vi "Determine_Meas_Analysis.vi"(1 "Pre Setup String":string, 2 "Analysis info Cluster In":T1[](array[typedef]) {"Kurt_u" format="%_3g"; "u^4" format="%_3g"; "u^3" format="%_3g"; "Sd Error in Variance" format="%_3g"; "u^2" format="%_3g"; "Sd Error in Mean" format="%_3g"; "U" format="%_3g"; "Sync Delay Time (s)" format="%.4f"; "Total Meas Time (s)" format="%_5g"; "Skew_u" format="%_3g"; "% u'/U" format="%_3g"}) -> (0 "Analysis info Cluster Out":T1[](array[typedef]) {"Kurt_u" format="%_3g"; "u^4" format="%_3g"; "u^3" format="%_3g"; "Sd Error in Variance" format="%_3g"; "u^2" format="%_3g"; "Sd Error in Mean" format="%_3g"; "U" format="%_3g"; "Sync Delay Time (s)" format="%.4f"; "Total Meas Time (s)" format="%_5g"; "Skew_u" format="%_3g"; "% u'/U" format="%_3g"})   [LabVIEW 2022 SP3]
uses:
  Globals/Meas_global.vi
  Controls/Inst_type.ctl
  Controls/Analysis_info_cluster.ctl
  Controls/Instrument_Array.ctl
  Acquisition/PWA/PWAtasksGLOBAL.vi
  7 Hole Probe pressures to UVW/7HP_Global.vi
  Acquisition/Device ID port info.ctl
  Controls/channelState.ctl
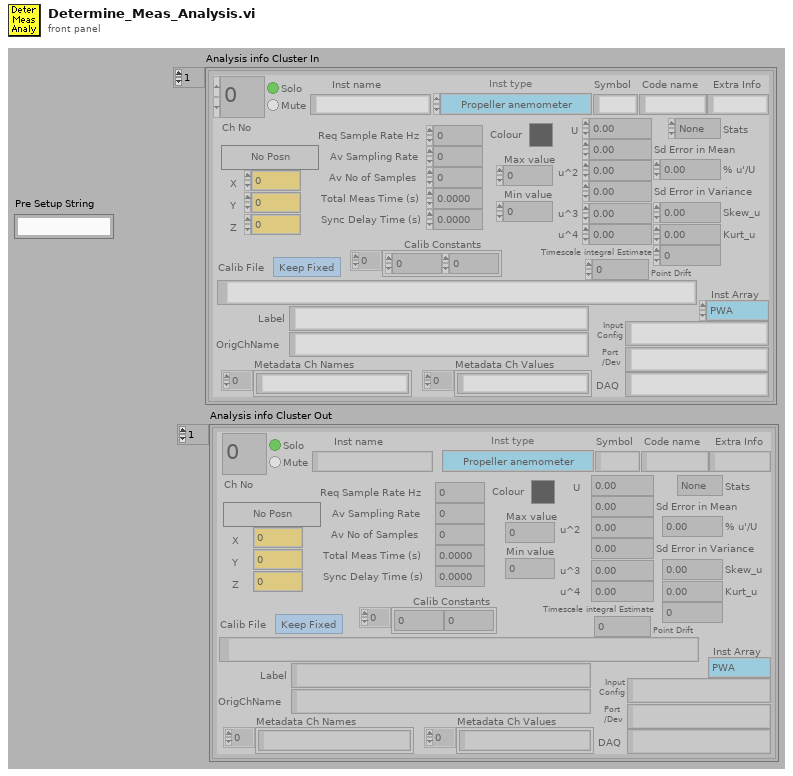
[diagram p1: front panel]
types:
  T1 = typedef "Analysis_info_cluster.ctl" = cluster{"Colour":u32, "Inst type":T2, "Inst name":string, "Symbol":string, "Code name":string, "Extra Info":string, "Inst Array":T3, "U":dbl, "u^2":dbl, "u^3":dbl, "u^4":dbl, "Skew_u":dbl, "Kurt_u":dbl, "Sd Error in Mean":dbl, "% u'/U":dbl, "X":dbl, "Y":dbl, "Z":dbl, "Timescale integral Estimate":dbl, "Sd Error in Variance":dbl, "Calib File":path, "Calib Constants":dbl[], "Output Position":bool, "Stats":enum16{"None", "Basic", "Full"}, "Av Sampling Rate":dbl, "Av No of Samples":dbl, "Total Meas Time (s)":dbl, "OrigChName":string, "Max value":dbl, "Min value":dbl, "Req Sample Rate Hz":dbl, "Sync Delay Time (s)":dbl, "Ch No":i16, "Device":string, "Use Latest Calib":bool, "Port":string, "Metadata Ch Names":string[], "Metadata Ch Values":string[], "Label":string, "chState":T4, "Point Drift":dbl, "inputConfig":string}
  T2 = typedef "Inst_type.ctl" = enum16{"Raw voltage", "Raw with zero offsetting", "Propeller anemometer", "Pressure Transducer", "Pitot-static tube", "Hot wire", "Cross wire 1", "Cross wire 2", "Generic Linear", "Generic Polynomial", "Generic BackPoly", "Fast FID", "Thermocouple", "Cold wire", "Pulsed Wire", "LDA Vel", "LDA Tran time", "LDA Arr time", "Microphone"}
  T3 = typedef "Instrument_Array.ctl" = enum16{"PWA", "LDA", "Analogue"}
  T4 = typedef "channelState.ctl" = enum32{"No Selection", "Solo", "Mute"}
  T5 = typedef "Post_Process.ctl" = enum16{"Take New Data", "Post Process Raw Data File"}
  T6 = cluster{"Pressure Ch Names":string[], "Pressure Index":i32[], "Metadata Index":i32[], "Port":string}[]
  T7 = typedef "Device ID port info.ctl" = cluster{"Ch No":i16[], "Req Sampling Rate":dbl[], "Port":string, "Index":i32[]}
  T8 = typedef "PWA_Data.ctl" = enum16{"No PWA Data", "One Ch PWA"}
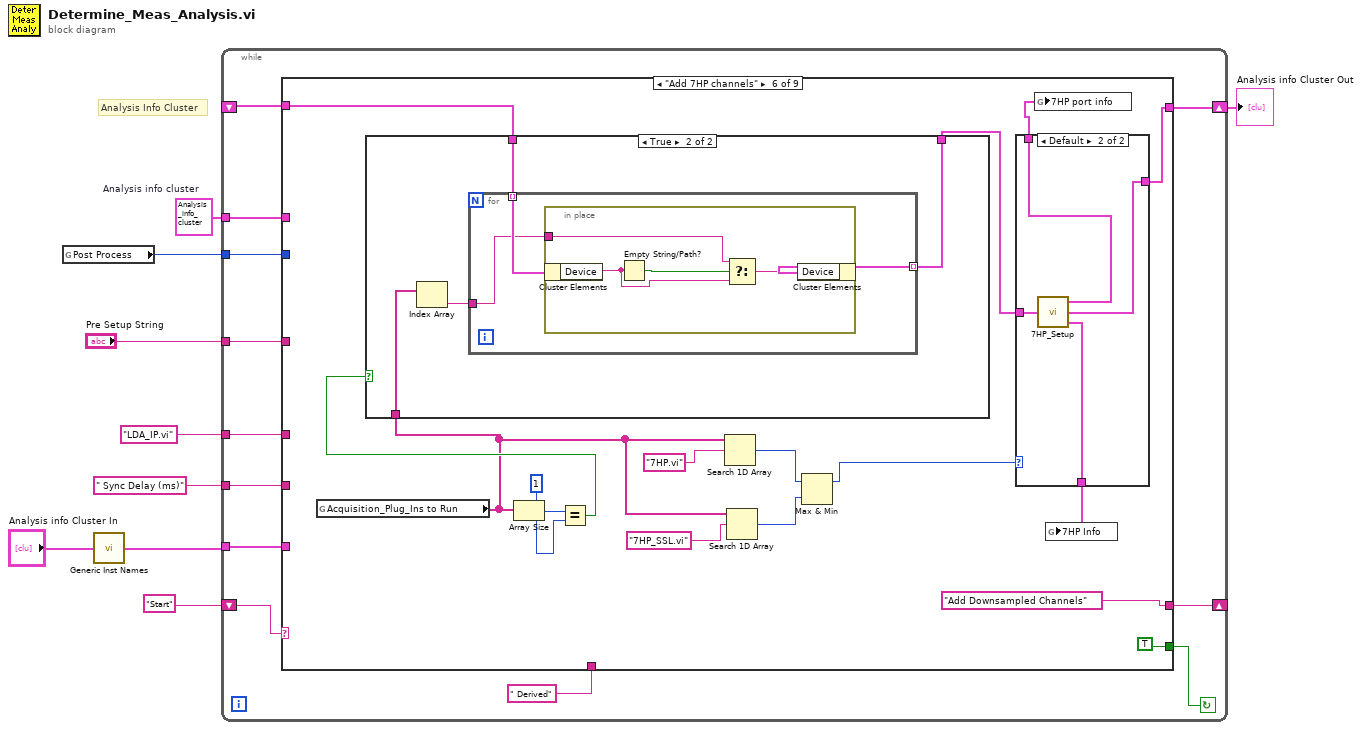
[diagram p0: block diagram]
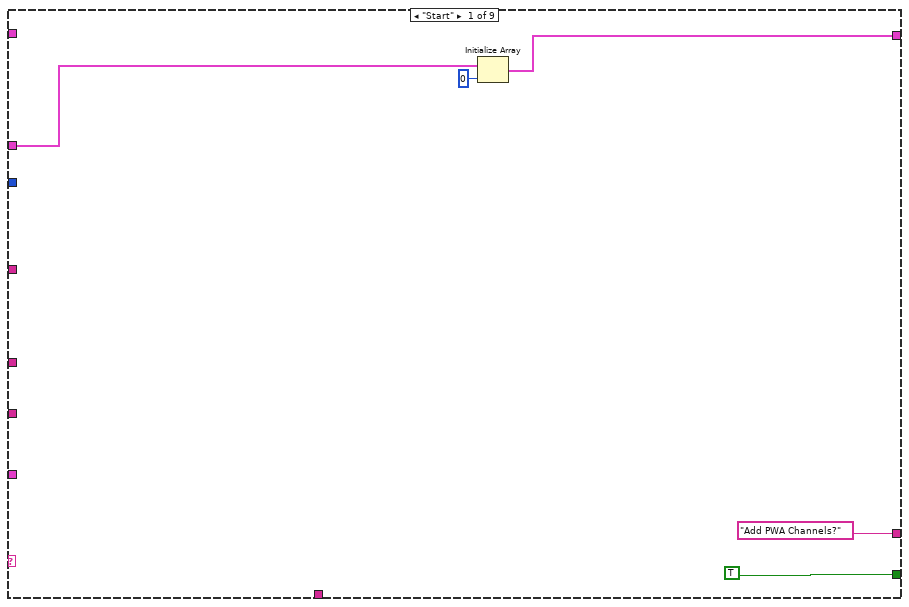
[diagram p2: hidden frame]
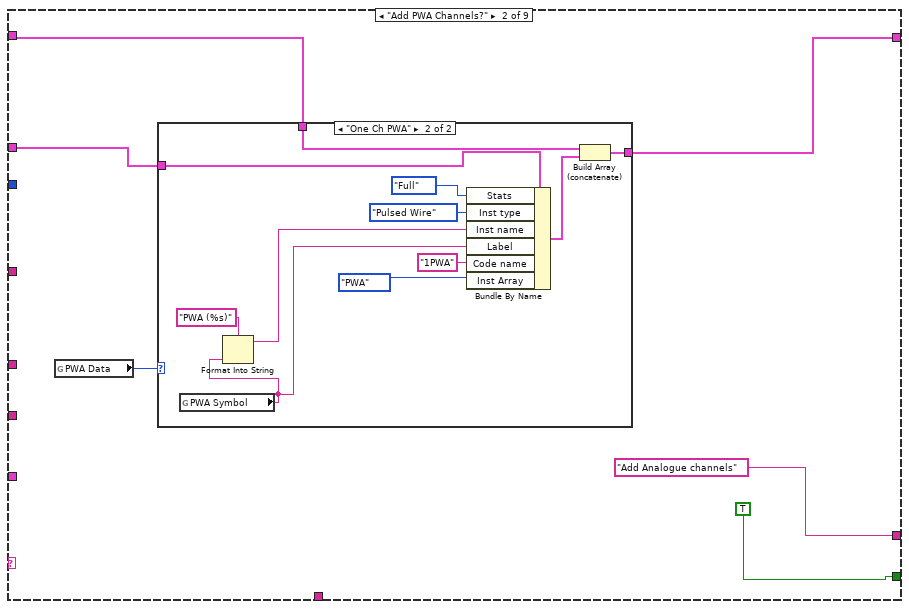
[diagram p3: hidden frame]
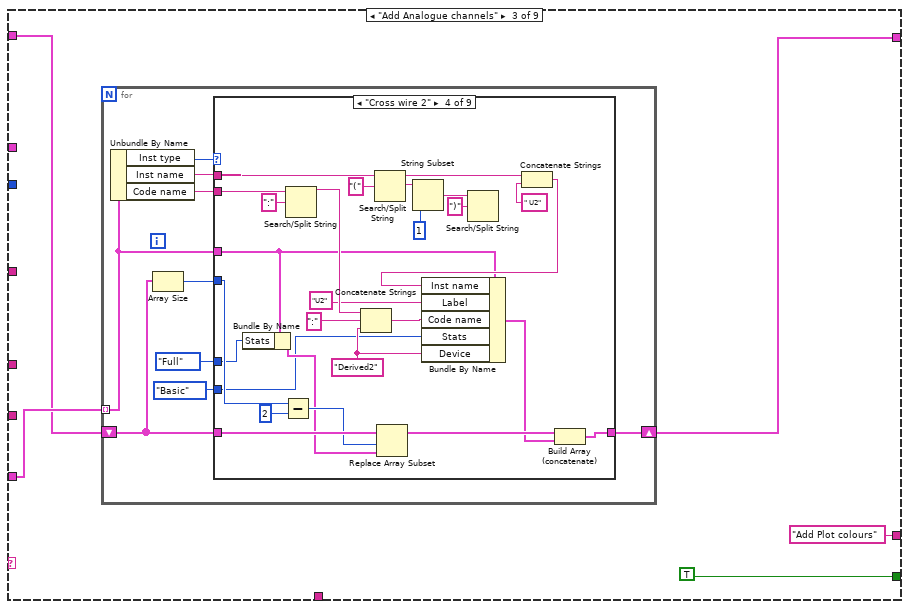
[diagram p5: hidden frame]
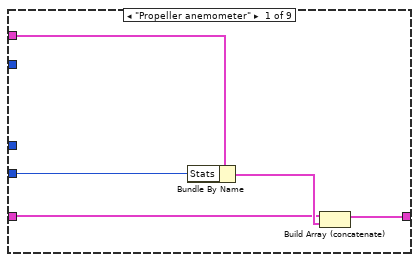
[diagram p6: hidden frame]
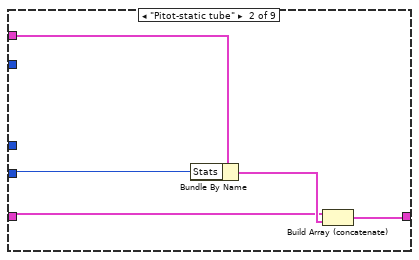
[diagram p7: hidden frame]
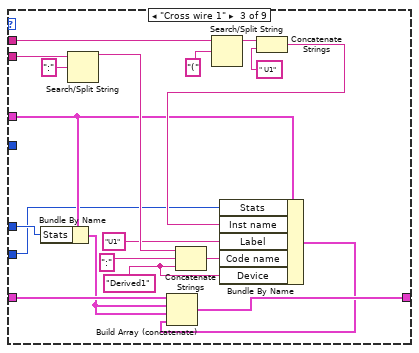
[diagram p8: hidden frame]
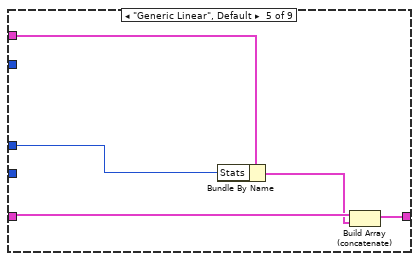
[diagram p9: hidden frame]
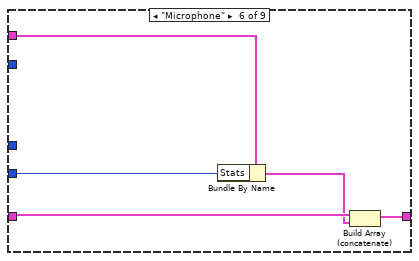
[diagram p10: hidden frame]
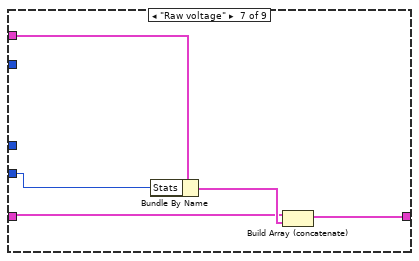
[diagram p11: hidden frame]
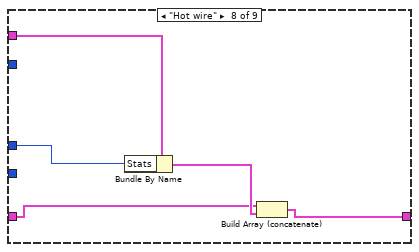
[diagram p12: hidden frame]
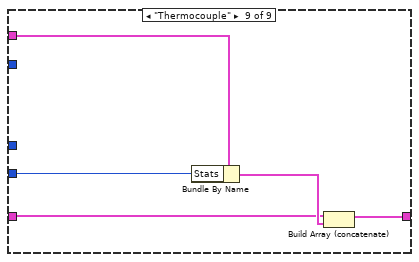
[diagram p13: hidden frame]
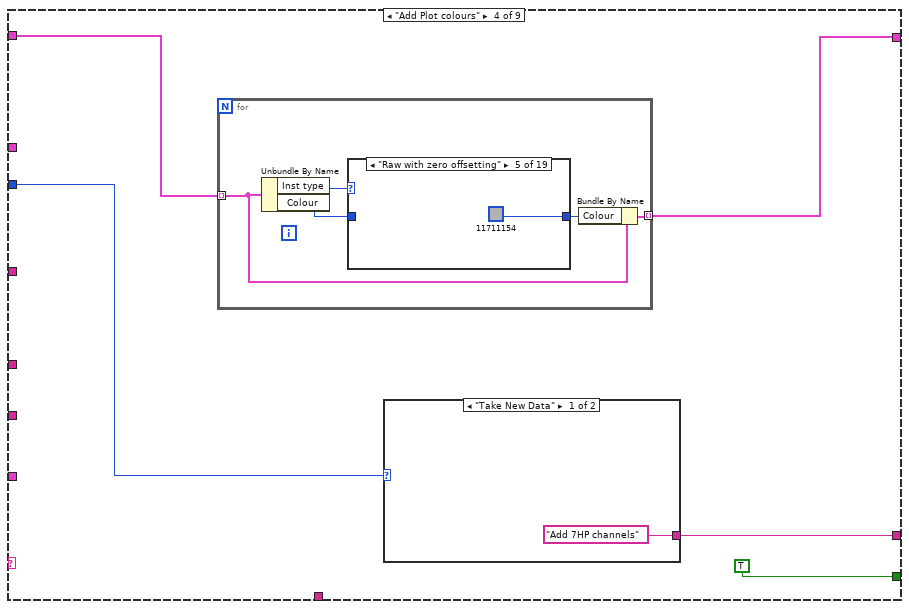
[diagram p14: hidden frame]
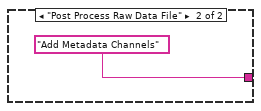
[diagram p15: hidden frame]
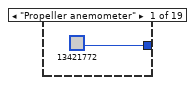
[diagram p16: hidden frame]
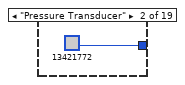
[diagram p17: hidden frame]
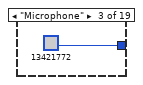
[diagram p18: hidden frame]
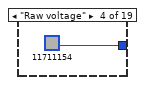
[diagram p19: hidden frame]
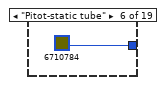
[diagram p20: hidden frame]
diagram:
  w9 = T1 {"Colour"=0, "Inst type"=enum."Pitot-static tube", "Inst name"="Manometer voltage", "Symbol"="U", "Code name"="", "Extra Info"="U", "Inst Array"=enum."PWA", "U"=0.0, "u^2"=0.0, "u^3"=0.0, "u^4"=0.0, "Skew_u"=0.0, "Kurt_u"=0.0, "Sd Error in Mean"=0.0, "% u'/U"=0.0, "X"=0.0, "Y"=0.0, "Z"=0.0, "Timescale integral Estimate"=0.0, "Sd Error in Variance"=0.0, "Calib File"=path "", "Calib Constants"=[], "Output Position"=FALSE, "Stats"=enum."None", "Av Sampling Rate"=0.0, "Av No of Samples"=0.0, "Total Meas Time (s)"=0.0, "OrigChName"="", "Max value"=0.0, "Min value"=0.0, "Req Sample Rate Hz"=0.0, "Sync Delay Time (s)"=0.0, "Ch No"=0, "Device"="", "Use Latest Calib"=FALSE, "Port"="", "Metadata Ch Names"=[], "Metadata Ch Values"=[], "Label"="", "chState"=enum."Solo", "Point Drift"=0.0, "inputConfig"=""}  # Analysis info cluster
  # "Analysis Info Cluster"
  n1 = global read "Meas_global.vi" "Post Process"() -> (w5:T5)
  n2 = call "Generic Inst Names.vi"("Analysis Info cluster"="Analysis info Cluster In") -> ("Analysis Info cluster out"=w1:T1[])  [unwired: 4 in]
  n3 = while {
    tunnel: w1 -> [w17]
    tunnel: w9 -> [w19]
    shift-left: _ -> [w18]
    shift-right: [w20] -> w7
    shift-right: [w16] -> _
    shift-left: "Start" -> [w15]
    tunnel: "Pre Setup String" -> [w14]
    tunnel: w5 -> [w13]
    tunnel: " Sync Delay (ms)" -> [w12]
    tunnel: "LDA_IP.vi" ("Device ID") -> [w11]
    stop <- w21 continue-if-true
    n4 = case shown="\"Add 7HP channels\"" w15 {
      selector: w15 -> [_ _ _ _ _ _ _ _ w285]
      tunnel: [TRUE TRUE TRUE TRUE TRUE TRUE TRUE FALSE FALSE] -> w21
      tunnel: [w24 w27 w48 w143 w174 w217 w247 w273 w287] -> w20
      tunnel: w19 -> [w23 w29 _ _ _ _ _ _ _]
      tunnel: w18 -> [_ w28 w45 w144 w175 w220 w245 w273 w287]
      tunnel: w17 -> [_ _ w46 _ _ _ _ _ _]
      tunnel: ["Add PWA Channels?" "Add Analogue channels" "Add Plot colours" w141 "Add 7HP channels" "Add Downsampled Channels" "End" "End" "End"] -> w16
      tunnel: w14 -> [_ _ _ _ w171 _ _ _ _]
      tunnel: w13 -> [_ _ _ w140 _ _ _ _ _]
      tunnel: w12 -> [_ _ _ _ _ _ _ _ _]
      tunnel: w11 -> [_ _ _ _ _ _ _ _ _]
      tunnel: " Derived" -> [_ _ _ _ _ _ w246 w270 _]
      frame "Start" {
        n5 = Initialize Array(w23, 0 ("Dimension Size")) -> (w24:T1[])
      }
      frame "Add PWA Channels?" {
        n6 = global read "Meas_global.vi" "PWA Data"() -> (w31:T8)
        n7 = case shown="\"One Ch PWA\"" w31 {
          tunnel: w29 -> [_ w44]
          tunnel: w28 -> [w33 w35]
          tunnel: [w33 w42] -> w27
          frame "No PWA Data" {
          }
          frame "One Ch PWA" {
            n8 = global read "PWAtasksGLOBAL.vi" "PWA Symbol"() -> (w36:string)
            n9 = Format Into String(format string="PWA (%s)", w36) -> (resulting string=w37:string)  [unwired: 2 in, 1 out]
            n10 = Bundle By Name(cluster=w44, "Stats"=enum16{"None", "Basic", "Full"}."Full", "Inst type"=Inst_type."Pulsed Wire", "Inst name"=w37, "Label"=w36, "Code name"="1PWA", "Inst Array"=Instrument_Array."PWA") -> (w43:T1)
            n11 = Build Array (concatenate)(w35, w43) -> (w42:T1[])
          }
        }
      }
      frame "Add Analogue channels" {
        n12 = for {
          tunnel: w46 -> [w57] mode=indexing
          shift-right: [w56] -> w48
          shift-left: w45 -> [w53]
          n13 = Unbundle By Name(w57) -> ("Inst type"=w58:T2, "Inst name"=w54:string, "Code name"=w55:string)
          n14 = Array Size(array=w53) -> (size(s)=w52:i32)
          n15 = case shown="\"Cross wire 2\"" w58 {
            tunnel: w54 -> [_ _ w78 w107 _ _ _ _ _]
            tunnel: w53 -> [w62 w66 w75 w96 w118 w123 w128 w131 w138]
            tunnel: w57 -> [w60 w65 w74 w105 w119 w124 w126 w133 w136]
            tunnel: [w61 w67 w77 w91 w116 w121 w127 w132 w137] -> w56
            tunnel: w55 -> [_ _ w76 w106 _ _ _ _ _]
            tunnel: w52 -> [_ _ _ w98 _ _ _ _ _]
            tunnel: enum16{"None", "Basic", "Full"}."Basic" ("Stats") -> [w59 w64 w69 w88 _ w120 w125 _ w135]
            tunnel: enum16{"None", "Basic", "Full"}."Full" ("Stats") -> [_ _ w70 w89 w115 _ _ w130 _]
            frame "Propeller anemometer" {
              n16 = Bundle By Name(cluster=w60, "Stats"=w59) -> (w63:T1)
              n17 = Build Array (concatenate)(w62, w63) -> (w61:T1[])
            }
            frame "Pitot-static tube" {
              n18 = Bundle By Name(cluster=w65, "Stats"=w64) -> (w68:T1)
              n19 = Build Array (concatenate)(w66, w68) -> (w67:T1[])
            }
            frame "Cross wire 1" {
              w71 = "Derived1"
              n20 = Bundle By Name(cluster=w74, "Stats"=w70) -> (w73:T1)
              n21 = Search/Split String(string=w76, search string/char (-)=":" ("search char (-)")) -> (substring before match=w81:string)  [unwired: 3 out]
              n22 = Concatenate Strings(w81, ":" ("search char (-)"), w71) -> (w82:string)
              n23 = Search/Split String(string=w78, search string/char (-)="(") -> (substring before match=w86:string)  [unwired: 3 out]
              n24 = Concatenate Strings(w86, " U1") -> (w85:string)
              n25 = Bundle By Name(cluster=w74, "Stats"=w69, "Inst name"=w85, "Label"="U1", "Code name"=w82, "Device"=w71) -> (w72:T1)
              n26 = Build Array (concatenate)(w75, w73, w73, w72) -> (w77:T1[])
            }
            frame "Cross wire 2" {
              w90 = "Derived2"
              n27 = Bundle By Name(cluster=w105, "Stats"=w89) -> (w94:T1)
              n28 = Subtract(x=w98, y=2) -> (x-y=w95:i32)
              n29 = Search/Split String(string=w106, search string/char (-)=":" ("search char (-)")) -> (substring before match=w110:string)  [unwired: 3 out]
              n30 = Concatenate Strings(w110, ":" ("search char (-)"), w90) -> (w111:string)
              n31 = Search/Split String(string=w107, search string/char (-)="(") -> (substring before match=w102:string, match + rest of string=w100:string)  [unwired: 2 out]
              n32 = Replace Array Subset(array=w96, new element=w94, index=w95) -> (w93:T1[])
              n33 = String Subset(string=w100, offset (0)=1) -> (substring=w99:string)  [unwired: 1 out]
              n34 = Search/Split String(string=w99, search string/char (-)=")") -> ()  [unwired: 4 out]
              n35 = Concatenate Strings(w102, " U2") -> (w114:string)
              n36 = Bundle By Name(cluster=w105, "Inst name"=w114, "Label"="U2", "Code name"=w111, "Stats"=w88, "Device"=w90) -> (w92:T1)
              n37 = Build Array (concatenate)(w93, w92) -> (w91:T1[])
            }
            frame "Generic Linear", Default {
              n38 = Bundle By Name(cluster=w119, "Stats"=w115) -> (w117:T1)
              n39 = Build Array (concatenate)(w118, w117) -> (w116:T1[])
            }
            frame "Microphone" {
              n40 = Bundle By Name(cluster=w124, "Stats"=w120) -> (w122:T1)
              n41 = Build Array (concatenate)(w123, w122) -> (w121:T1[])
            }
            frame "Raw voltage" {
              n42 = Bundle By Name(cluster=w126, "Stats"=w125) -> (w129:T1)
              n43 = Build Array (concatenate)(w128, w129) -> (w127:T1[])
            }
            frame "Hot wire" {
              n44 = Bundle By Name(cluster=w133, "Stats"=w130) -> (w134:T1)
              n45 = Build Array (concatenate)(w131, w134) -> (w132:T1[])
            }
            frame "Thermocouple" {
              n46 = Bundle By Name(cluster=w136, "Stats"=w135) -> (w139:T1)
              n47 = Build Array (concatenate)(w138, w139) -> (w137:T1[])
            }
          }
        }
      }
      frame "Add Plot colours" {
        n48 = for {
          tunnel: [w149] -> w143 mode=indexing
          tunnel: w144 -> [w147] mode=indexing
          n49 = Unbundle By Name(w147) -> ("Inst type"=w151:T2, "Colour"=w148:u32)
          n50 = case shown="\"Raw with zero offsetting\"" w151 {
            tunnel: [u32 13421772 u32 13421772 u32 13421772 u32 11711154 u32 11711154 u32 6710784 u32 16724736 u32 13382400 u32 10040217 u32 16711935 u32 16711935 u32 16711935 u32 65535 u32 16776960 u32 10027263 u32 10027263 w168 u32 65280 u32 65280] -> w150
            tunnel: w148 -> [_ _ _ _ _ _ _ _ _ _ _ _ _ _ _ _ w168 _ _]
            frame "Propeller anemometer" {
            }
            frame "Pressure Transducer" {
            }
            frame "Microphone" {
            }
            frame "Raw voltage" {
            }
            frame "Raw with zero offsetting" {
            }
            frame "Pitot-static tube" {
            }
            frame "Hot wire" {
            }
            frame "Cross wire 1" {
            }
            frame "Cross wire 2" {
            }
            frame "Generic Linear" {
            }
            frame "Generic Polynomial" {
            }
            frame "Generic BackPoly" {
            }
            frame "Fast FID" {
            }
            frame "Thermocouple" {
            }
            frame "Cold wire" {
            }
            frame "Pulsed Wire" {
            }
            frame "LDA Vel" {
            }
            frame "LDA Tran time" {
            }
            frame "LDA Arr time" {
            }
          }
          n51 = Bundle By Name(cluster=w147, "Colour"=w150) -> (w149:T1)
        }
        n52 = case shown="\"Take New Data\"" w140 {
          tunnel: ["Add 7HP channels" "Add Metadata Channels"] -> w141
          frame "Take New Data" {
          }
          frame "Post Process Raw Data File" {
          }
        }
      }
      frame "Add Metadata Channels" {
        n53 = for {
          tunnel: [w176] -> w174 mode=indexing
          tunnel: w175 -> [w179] mode=indexing
          tunnel: w171 -> [w180]
          i -> [w182]
          n54 = Format Into String(format string="Metadata Ch Names for Index_%3d", w182) -> (resulting string=w184:string)  [unwired: 2 in, 1 out]
          n55 = call "Get_Characters_from_string.vi"("Show Dialog?"=FALSE, "Input string"=w180, "Variable name"=w184) -> ("Status"=w183:enum16{"Char in string", "Char not in string"}, "Value"=w181:string)
          n56 = case shown="\"Char not in string\"" w183 {
            tunnel: w182 -> [w196 _]
            tunnel: w181 -> [w195 _]
            tunnel: [w189 w208] -> w178
            tunnel: [w188 w208] -> w177
            tunnel: w180 -> [w193 _]
            frame "Char in string" {
              n57 = Format Into String(format string="Metadata Ch Values for Index_%3d", w196) -> (resulting string=w194:string)  [unwired: 2 in, 1 out]
              n58 = call "Get_array_values_fr_String.vi"("String Value"=w195) -> ("String array"=w190:string[])  [unwired: 1 out]
              n59 = call "Get_Characters_from_string.vi"("Input string"=w193, "Variable name"=w194) -> ("Value"=w192:string)  [unwired: 1 in, 1 out]
              n60 = call "Get_array_values_fr_String.vi"("String Value"=w192) -> ("String array"=w187:string[])  [unwired: 1 out]
              n61 = for {
                shift-right: [w203] -> w189
                shift-left: string[] [] -> [w202]
                tunnel: w190 -> [w200] mode=indexing
                tunnel: [w201] -> w188 mode=indexing if=w198
                tunnel: w187 -> [w201] mode=indexing
                n62 = Search 1D Array(1D array=w202, element=w200) -> (index of element=w199:i32)  [unwired: 1 in]
                n63 = Less Than 0?(x=w199) -> (x < 0?=w198:bool)
                n64 = case shown="True" w198 {
                  tunnel: w200 -> [_ w207]
                  tunnel: [w204 w206] -> w203
                  tunnel: w202 -> [w204 w205]
                  frame False {
                  }
                  frame True {
                    n65 = Build Array (concatenate)(w205, w207) -> (w206:string[])
                  }
                }
              }
            }
            frame "Char not in string" {
              w208 = string[] [] ("String array")
            }
          }
          n66 = call "Update Metadata channels.vi"("Metadata Values"=w177, "Metadata Names"=w178, "Analysis info Cluster in"=w179) -> ("Analysis info Cluster out"=w176:T1)
        }
      }
      frame "Add 7HP channels" {
        n67 = global read "Meas_global.vi" "Acquisition_Plug_Ins to Run"() -> (w213:string[])
        n68 = Array Size(array=w213) -> (size(s)=w223:i32)
        n69 = Equal?(x=w223, y=1) -> (x = y?=w221:bool)
        n70 = case shown="True" w221 {
          tunnel: w220 -> [w232 w236]
          tunnel: [w232 w235] -> w218
          tunnel: w213 -> [_ w234]
          frame False {
          }
          frame True {
            n71 = Index Array(array=w234) -> (element=w233:string)  [unwired: 1 in]
            n72 = for {
              tunnel: w236 -> [w239] mode=indexing
              tunnel: [w238] -> w235 mode=indexing
              tunnel: w233 -> [w237]
              n73 = in-place {
                in-place-border: w237 -> [w242]
                n74 = in-place-cluster #1(w239) -> ("Device"=w241:string)
                n75 = Empty String/Path?(string/path=w241) -> (empty?=w243:bool)
                n76 = Select(t=w242, s=w243, f=w241) -> (s? t:f=w240:string)
                n77 = in-place-cluster #1("Device"=w240) -> (w238:T1)
              }
            }
          }
        }
        n78 = Search 1D Array(1D array=w213, element="7HP.vi") -> (index of element=w212:i32)  [unwired: 1 in]
        n79 = Search 1D Array(1D array=w213, element="7HP_SSL.vi") -> (index of element=w211:i32)  [unwired: 1 in]
        n80 = Max & Min(x=w212, y=w211) -> (max(x,y)=w210:i32)  [unwired: 1 out]
        n81 = case shown="Default" w210 {
          tunnel: w218 -> [w227 w231]
          tunnel: [w227 w230] -> w217
          tunnel: [T6 [] ("7HP Info") w229] -> w216
          tunnel: [T7[] [] ("Device port info") w228] -> w215
          frame -1 {
          }
          frame Default {
            n82 = call "7HP_Setup.vi"("Analysis Info cluster In"=w231) -> ("Device port info"=w228:T7[], "Analysis Info cluster Out"=w230:T1[], "7HP Info"=w229:T6)  [unwired: 4 in]
          }
        }
        n83 = global write "7HP_Global.vi" "7HP port info"(w215) -> ()
        n84 = global write "7HP_Global.vi" "7HP Info"(w216) -> ()
      }
      frame "Add Downsampled Channels" {
        n85 = for {
          tunnel: w246 -> [w254]
          tunnel: w245 -> [w253] mode=indexing
          tunnel: [w257] -> w244 mode=indexing if=w256
          n86 = Unbundle By Name(w253) -> ("Code name"=w255:string)
          n87 = call "Meas Channels to Average.vi"("Analysis_info_cluster"=w253) -> ("Create Av Channel"=w251:bool, "Label"=w250:string, "Av Inst name"=w252:string)  [unwired: 7 in, 1 out]
          n88 = case shown="True" w251 {
            tunnel: w253 -> [w259 w268]
            tunnel: [w259 w267] -> w257
            tunnel: [FALSE TRUE] -> w256
            tunnel: w255 -> [_ w265]
            tunnel: w254 -> [_ w263]
            tunnel: w252 -> [_ w261]
            tunnel: w250 -> [_ w260]
            frame False {
            }
            frame True {
              n89 = Concatenate Strings(w265, w263) -> (w264:string)
              n90 = Bundle By Name(cluster=w268, "Inst name"=w261, "Label"=w260, "Code name"=w264, "Device"=w263, "Req Sample Rate Hz"=10.0) -> (w267:T1)
            }
          }
        }
        n91 = Build Array (concatenate)(w245, w244) -> (w247:T1[])
      }
      frame "End" {
        # "Changed from \"=\" as X-wire additional are called \"Derived1\" and \"Derived2\" TCRL 2022-05-09"
        n92 = call <vilib>:"Trim Whitespace.vi"("string"=w270) -> ("trimmed string"=w269:string)  [unwired: 1 in]
        n93 = for {
          tunnel: w273 -> [w284] mode=indexing
          tunnel: [w283] -> w272 mode=indexing if=w278
          tunnel: w269 -> [w282]
          n94 = Unbundle By Name(w284) -> ("chState"=w280:T4, "Device"=w283:string)
          n95 = Not Equal?(x=channelState."Mute" ("chState"), y=w280) -> (x != y?=w276:bool)
          n96 = Match Pattern(string=w283, regular expression=w282) -> (offset past match=w281:i32)  [unwired: 1 in, 3 out]
          n97 = Less Than 0?(x=w281) -> (x < 0?=w277:bool)
          n98 = And(x=w276, y=w277) -> (x .and. y?=w278:bool)
        }
        n99 = call "Analyse_string_array.vi"("String array"=w272) -> ("Unique strings"=w271:string[])  [unwired: 1 in, 1 out]
        n100 = global write "Meas_global.vi" "Acquisition_Plug_Ins to Run"(w271) -> ()
      }
      frame "No Match", Default {
        n101 = call "Case not matched.vi"("Case Name not Matched"=w285) -> ()
      }
    }
  }
  "Analysis info Cluster Out" <- w7
